vi "DrumSequence_Execute.vi"(6 "Pass_Through_Time":dbl=-1.0 format="%33.4f", 8 "Cancel Time Sec":dbl, 9 "Step Times Sec":dbl[](array[numeric]), 10 "Cancel":bool, 11 "Initiate":bool) -> (0 "Error":bool, 1 "Ready":bool, 2 "Seq  Active":bool, 3 "Step Number":T1=enum."Initialize")   [LabVIEW 2019, in "Trajectory_Library.lvlib"]
doc: "Implements a simplified state machine similar to a mechanical / electrical drum sequencer. When the Drum Sequencer is \"Ready\" and the \"Initiate\" input becomes TRUE,, the drum sequences through its set of steps from 1 to N. After each Step is executed it is followed by a wait. During the wait the Step output indicates \"Do Nothing\". The number of Steps is determined by the number of elements in the \"Step Times\" input array. Once all the steps have been executed, the Drum Sequencer cycles bac to wait for another initiate. \n\nThere is a Cancel input that interrupts the sequence, executes the Cancel Step, performs the cancel wait, and then returns to wait for an Initiate action. \n\nIf any of the Step Times, or Cancel times are negative, or there more than 32 steps, or less than 1 step an error is signaled. The drum sequencer selects the error state and stays there.\n\nInputs:\n\nOutputs:"
uses:
  Trajectory_Library.lvlib
  Enum/DrumSequence_State_Enum.ctl
  Enum/DrumSequence_Step_Enum.ctl
panel:
  # "Time to wait\nafter executing\nstep"
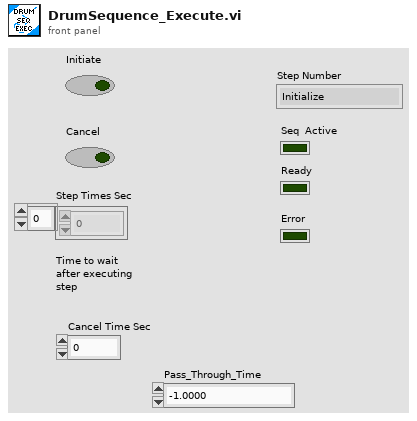
[diagram p1: front panel]
types:
  T1 = typedef "Trajectory_Library.lvlib/DrumSequence_Step_Enum.ctl" = enum16{"Do Nothing", "Step 1", "Step 2", "Step 3", "Step 4", "Step 5", "Step 6", "Step 7", "Step 8", "Step 9", "Step 10", "Step 11", "Step 12", "Step 13", "Step 14", "Step 15", "Step 16", "Step 17", "Step 18", "Step 19", "Step 20", "Step 21", "Step 22", "Step 23", "Step 24", "Step 25", "Step 26", "Step 27", "Step 28", "Step 29", "Step 30", "Step 31", "Step 32", "Cancel", "Initialize", "Error"}
  T2 = typedef "Trajectory_Library.lvlib/DrumSequence_State_Enum.ctl" = enum16{"Initialize", "Ready", "First Step", "Step Wait", "Next State", "Cancel", "Cancel Wait", "Error", "Error Loop"}
  T3 = typedef "Trajectory_Library.lvlib/TIMER.ctl" = cluster{"StartTime":dbl, "Accumulated TIme":dbl, "Running":bool, "semaphore":T4}
  T4 = typedef "Semaphore RefNum" = refnum<k1>
  T5 = typedef "DrumSequence_State_Enum.ctl" = enum16{"Initialize", "Ready", "First Step", "Step Wait", "Next State", "Cancel", "Cancel Wait", "Error", "Error Loop"}
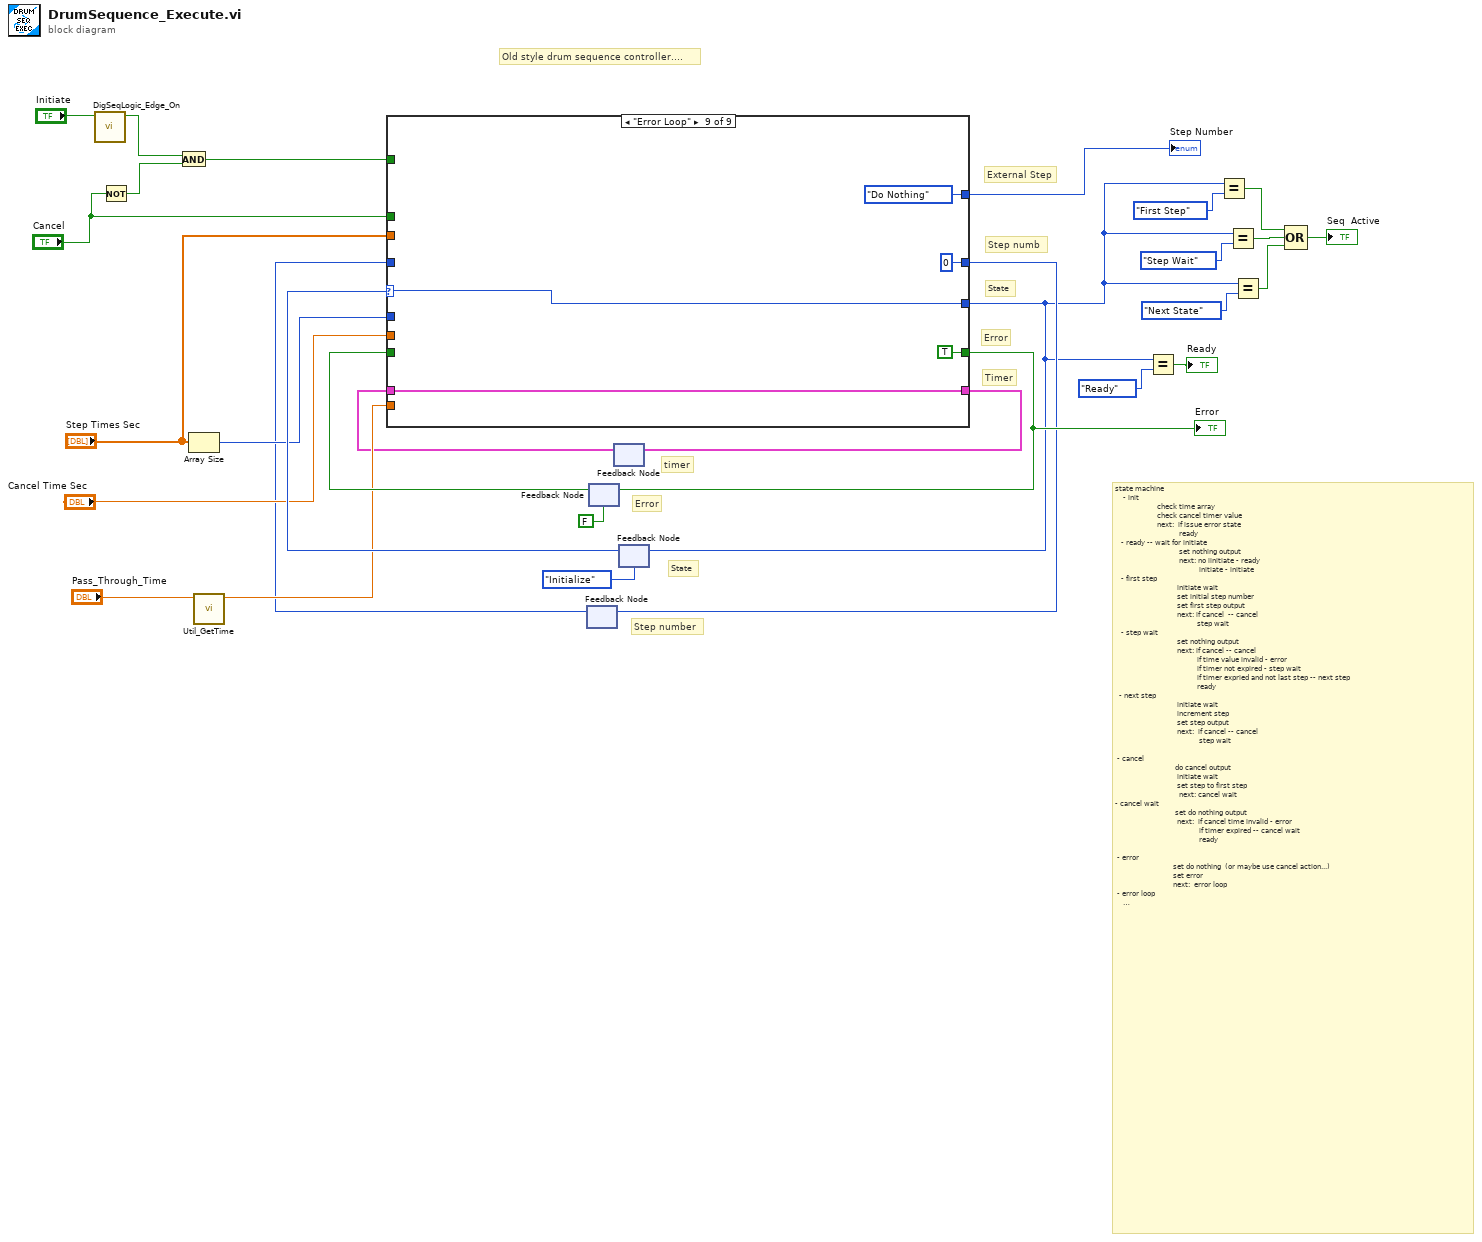
[diagram p0: block diagram]
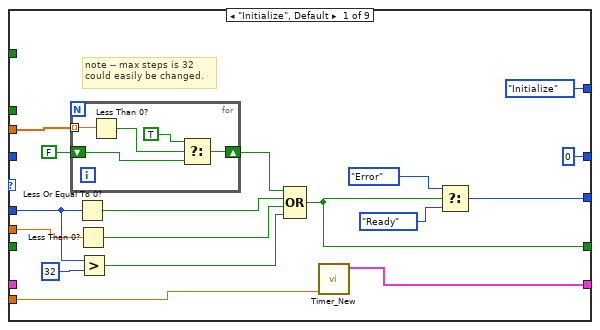
[diagram p2: hidden frame]
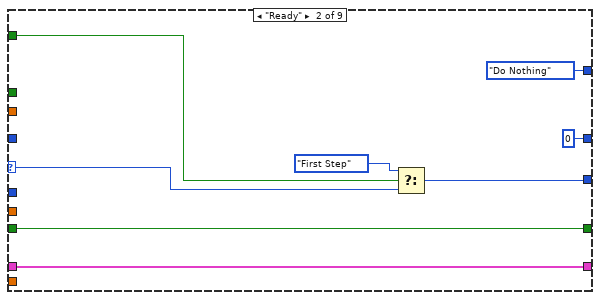
[diagram p3: hidden frame]
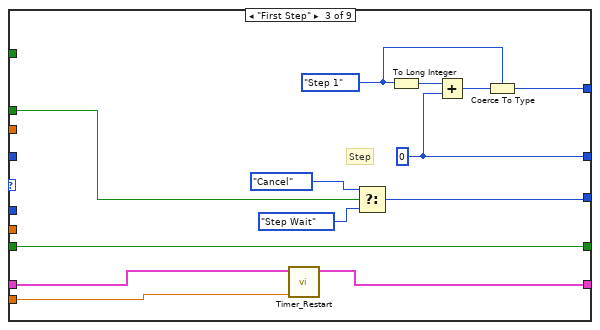
[diagram p4: hidden frame]
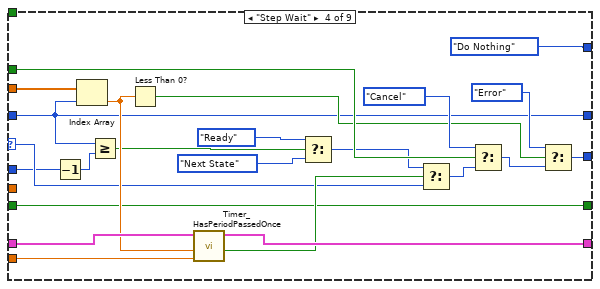
[diagram p5: hidden frame]
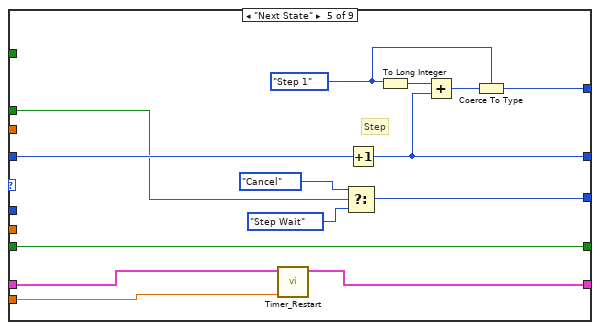
[diagram p6: hidden frame]
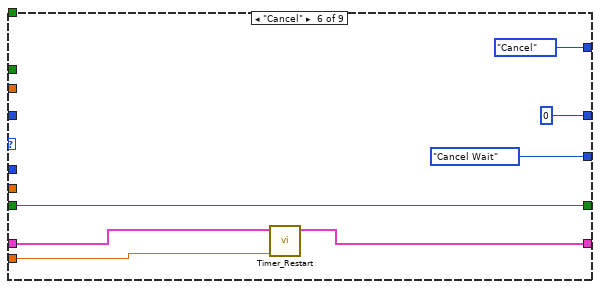
[diagram p7: hidden frame]
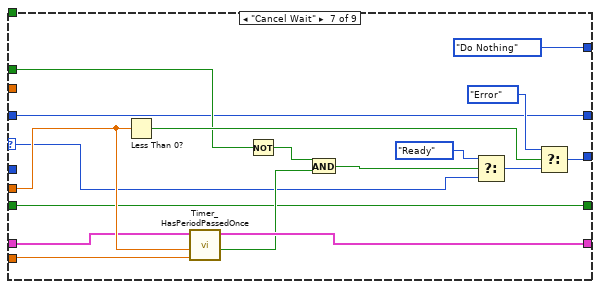
[diagram p8: hidden frame]
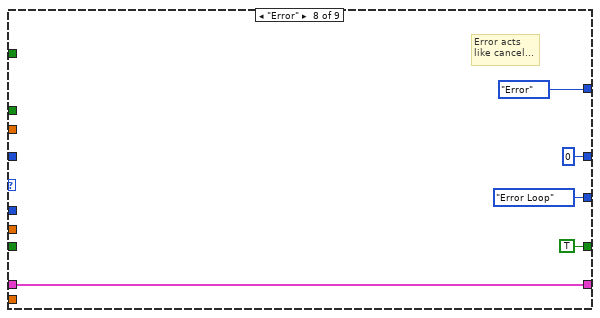
[diagram p9: hidden frame]
diagram:
  # "Old style drum sequence controller...."
  # "Step number"
  # "State"
  # "Step numb"
  # "timer"
  # "Timer"
  # "Error"
  # "State"
  # "External Step"
  # "Error"
  # "state machine\n    - init\n                     check time array\n                     check cancel timer value\n                     next:  if issue error state\n                                ready\n   - ready -- wait for initiate\n                                set nothing output\n                                next: no iinitiate - ready\n                                          initiate - initiate\n   - first step \n                               initiate wait\n                               set initial step number\n                               set first step output\n                               next: if cancel  -- cancel\n                                         step wait\n   - step wait \n                               set nothing output\n                               next: if cancel -- cancel\n                                         if time value invalid - error\n                                         if timer not expired - step wait\n                                         if timer expried and not last step -- next step\n                                         ready\n  - next step\n                               initiate wait\n                               increment step\n                               set step output\n                               next:  if cancel -- cancel\n                                          step wait\n\n - cancel\n                              do cancel output\n                               initiate wait\n                               set step to first step\n                                next: cancel wait\n- cancel wait\n                              set do nothing output\n                               next:  if cancel time invalid - error\n                                          if timer expired -- cancel wait\n                                          ready\n\n - error\n                             set do nothing  (or maybe use cancel action...)\n                             set error\n                             next:  error loop\n - error loop\n                             set do nothing\n                             set error\n                             next: error loop"
  n1 = call "DigSeqLogic_Edge_On.vi"("Input"="Initiate") -> ("On Edge"=w28:bool)  [unwired: 10 in]
  n2 = Not(x="Cancel") -> (.not. x?=w30:bool)
  n3 = And(x=w28, y=w30) -> (x .and. y?=w17:bool)
  n4 = Array Size(array="Step Times Sec") -> (size(s)=w25:i32)
  n5 = call "Util_GetTime.vi"("Pass_Through_Time"="Pass_Through_Time") -> ("FPGA_Time_Seconds"=w18:dbl)  [unwired: 8 in, 2 out]
  n6 = feedback #1() -> (w11:i32)  [unwired: 1 in]
  n7 = feedback #2(FALSE) -> (w20:bool)
  n8 = feedback #3() -> (w10:T3)  [unwired: 1 in]
  n9 = feedback #4(DrumSequence_State_Enum."Initialize") -> (w26:T5)
  n10 = case shown="\"Error Loop\"" w26 {
    selector: w26 -> [_ w57 _ w77 _ _ w119 _ w143]
    tunnel: w25 -> [w35 _ _ w75 _ _ _ _ _]
    tunnel: "Step Times Sec" -> [w46 _ _ w86 _ _ _ _ _]
    tunnel: "Cancel Time Sec" -> [w45 _ _ _ _ _ w131 _ _]
    tunnel: [w41 w56 w62 w78 w101 w113 w120 TRUE TRUE] -> w21
    tunnel: w20 -> [_ w56 w62 w78 w101 w113 w120 _ _]
    tunnel: [w38 w58 w63 w83 w103 DrumSequence_State_Enum."Cancel Wait" w124 DrumSequence_State_Enum."Error Loop" w143] -> w2
    tunnel: [w37 w55 w67 w94 w98 w114 w128 w137 w141] -> w14
    tunnel: w18 -> [w36 _ w69 w95 w100 w115 w129 _ _]
    tunnel: [DrumSequence_Step_Enum."Initialize" ("Step Number") DrumSequence_Step_Enum."Do Nothing" ("Step Number") w71 DrumSequence_Step_Enum."Do Nothing" ("Step Number") w104 DrumSequence_Step_Enum."Cancel" ("Step Number") DrumSequence_Step_Enum."Do Nothing" ("Step Number") DrumSequence_Step_Enum."Error" ("Step Number") DrumSequence_Step_Enum."Do Nothing" ("Step Number")] -> w1
    tunnel: w17 -> [_ w60 _ _ _ _ _ _ _]
    tunnel: [0 0 w70 w80 w105 0 w122 0 0] -> w12
    tunnel: "Cancel" -> [_ _ w66 w91 w102 _ w125 _ _]
    tunnel: w11 -> [_ _ _ w80 w106 _ w122 _ _]
    tunnel: w10 -> [_ w55 w68 w96 w99 w116 w130 w137 w141]
    frame "Initialize", Default {
      # "note -- max steps is 32\ncould easily be changed."
      n11 = for {
        shift-right: [w51] -> w44
        shift-left: FALSE -> [w50]
        tunnel: w46 -> [w52] mode=indexing
        n12 = Less Than 0?(x=w52) -> (x < 0?=w48:bool)
        n13 = Select(t=TRUE, s=w48, f=w50) -> (s? t:f=w51:bool)
      }
      n14 = Less Or Equal To 0?(x=w35) -> (x <= 0?=w43:bool)
      n15 = Less Than 0?(x=w45) -> (x < 0?=w42:bool)
      n16 = Greater?(x=w35, y=32) -> (0:w33:bool)
      n17 = Compound Arithmetic op=OR(w44, w43, w42, w33) -> (w41:bool)
      n18 = call "Timer_New.vi"("Pass_Through_Time"=w36) -> ("TIMER"=w37:T3)  [unwired: 10 in]
      n19 = Select(t=DrumSequence_State_Enum."Error", s=w41, f=DrumSequence_State_Enum."Ready") -> (s? t:f=w38:T2)
    }
    frame "Ready" {
      n20 = Select(t=DrumSequence_State_Enum."First Step", s=w60, f=w57) -> (s? t:f=w58:T5)
    }
    frame "First Step" {
      w61 = DrumSequence_Step_Enum."Step 1" ("Step Number")
      w70 = 0
      # "Step"
      n21 = call "Timer_Restart.vi"("Pass_Through_Time"=w69, "in Timer"=w68) -> ("out Timer"=w67:T3)  [unwired: 9 in]
      n22 = Select(t=DrumSequence_State_Enum."Cancel", s=w66, f=DrumSequence_State_Enum."Step Wait") -> (s? t:f=w63:T2)
      n23 = To Long Integer(number=w61) -> (32bit integer=w73:i32)
      n24 = Add(x=w73, y=w70) -> (x+y=w72:i32)
      n25 = Coerce To Type(0:w72, 1:w61) -> (2:w71:T1)
    }
    frame "Step Wait" {
      n26 = Decrement(x=w75) -> (x-1=w76:i32)
      n27 = Index Array(array=w86, index=w80) -> (element=w85:dbl)
      n28 = Greater Or Equal?(x=w80, y=w76) -> (x >= y?=w79:bool)
      n29 = Less Than 0?(x=w85) -> (x < 0?=w81:bool)
      n30 = call "Timer_HasPeriodPassedOnce.vi"("Pass_Through_Time"=w95, "Period"=w85, "in Timer"=w96) -> ("Expired"=w87:bool, "out Timer"=w94:T3)  [unwired: 6 in, 1 out]
      n31 = Select(t=DrumSequence_State_Enum."Ready", s=w79, f=DrumSequence_State_Enum."Next State") -> (s? t:f=w88:T2)
      n32 = Select(t=w88, s=w87, f=w77) -> (s? t:f=w92:T5)
      n33 = Select(t=DrumSequence_State_Enum."Cancel", s=w91, f=w92) -> (s? t:f=w82:T5)
      n34 = Select(t=DrumSequence_State_Enum."Error", s=w81, f=w82) -> (s? t:f=w83:T5)
    }
    frame "Next State" {
      w97 = DrumSequence_Step_Enum."Step 1" ("Step Number")
      # "Step"
      n35 = call "Timer_Restart.vi"("Pass_Through_Time"=w100, "in Timer"=w99) -> ("out Timer"=w98:T3)  [unwired: 9 in]
      n36 = Select(t=DrumSequence_State_Enum."Cancel", s=w102, f=DrumSequence_State_Enum."Step Wait") -> (s? t:f=w103:T2)
      n37 = Increment(x=w106) -> (x+1=w105:i32)
      n38 = To Long Integer(number=w97) -> (32bit integer=w110:i32)
      n39 = Add(x=w110, y=w105) -> (x+y=w109:i32)
      n40 = Coerce To Type(0:w109, 1:w97) -> (2:w104:T1)
    }
    frame "Cancel" {
      n41 = call "Timer_Restart.vi"("Pass_Through_Time"=w115, "in Timer"=w116) -> ("out Timer"=w114:T3)  [unwired: 9 in]
    }
    frame "Cancel Wait" {
      n42 = Less Than 0?(x=w131) -> (x < 0?=w132:bool)
      n43 = call "Timer_HasPeriodPassedOnce.vi"("Pass_Through_Time"=w129, "Period"=w131, "in Timer"=w130) -> ("Expired"=w127:bool, "out Timer"=w128:T3)  [unwired: 6 in, 1 out]
      n44 = Not(x=w125) -> (.not. x?=w126:bool)
      n45 = And(x=w126, y=w127) -> (x .and. y?=w121:bool)
      n46 = Select(t=DrumSequence_State_Enum."Ready", s=w121, f=w119) -> (s? t:f=w133:T5)
      n47 = Select(t=DrumSequence_State_Enum."Error", s=w132, f=w133) -> (s? t:f=w124:T5)
    }
    frame "Error" {
      # "Error acts\nlike cancel..."
    }
    frame "Error Loop" {
    }
  }
  "Error" <- w21
  "Step Number" <- w1
  n48 = feedback-in #1(w12) -> ()
  n49 = feedback-in #2(w21) -> ()
  n50 = feedback-in #3(w14) -> ()
  n51 = feedback-in #4(w2) -> ()
  n52 = Equal?(x=w2, y=DrumSequence_State_Enum."Ready") -> (x = y?=→"Ready":bool)
  n53 = Equal?(x=w2, y=DrumSequence_State_Enum."First Step") -> (x = y?=w6:bool)
  n54 = Equal?(x=w2, y=DrumSequence_State_Enum."Step Wait") -> (x = y?=w5:bool)
  n55 = Equal?(x=w2, y=DrumSequence_State_Enum."Next State") -> (x = y?=w4:bool)
  n56 = Compound Arithmetic op=OR(w6, w5, w4) -> (→"Seq  Active":bool)
